vi "MOVE_ELEVATOR_TO_TARGET.vi"(10 "argv":string[](array[string]), 11 "args":u8) -> ()   [LabVIEW 2014]
uses:
  Robot Global Data.vi
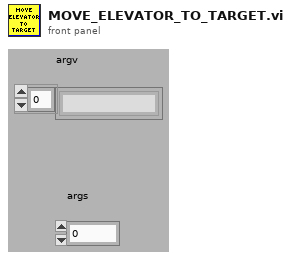
[diagram p1: front panel]
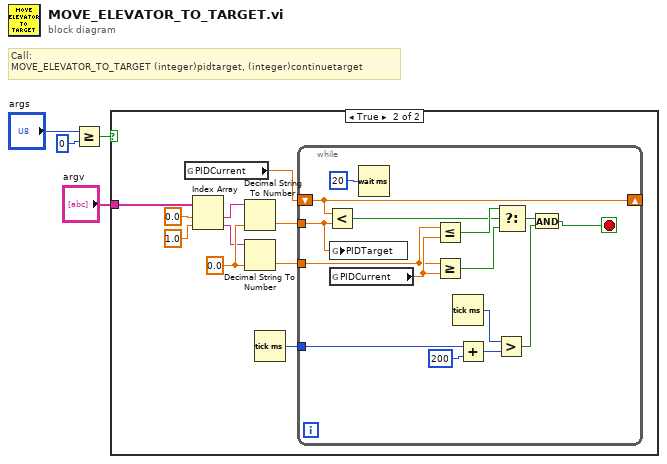
[diagram p0: block diagram]
diagram:
  # "Call:\nMOVE_ELEVATOR_TO_TARGET (integer)pidtarget, (integer)continuetarget"
  n1 = Greater Or Equal?(x="args", y=u8 0) -> (x >= y?=w4:bool)
  n2 = case shown="True" w4 {
    tunnel: "argv" -> [_ w11]
    frame False {
    }
    frame True {
      w6 = 0.0
      n3 = global read "OriginalPIDCurrent" "PIDCurrent"() -> (w13:dbl)
      n4 = Index Array(array=w11, index #1=0.0 ("default (0 I32)"), index #2=1.0 ("default (0 I32)")) -> (element #1=w9:string, element #2=w5:string)
      n5 = Decimal String To Number(string=w9, default (0L)=w6) -> (number=w8:dbl)  [unwired: 1 in, 1 out]
      n6 = Decimal String To Number(string=w5, default (0L)=w6) -> (number=w7:dbl)  [unwired: 1 in, 1 out]
      n7 = Tick Count (ms)() -> (millisecond timer value=w14:u32)
      n8 = while {
        tunnel: w8 -> [w19]
        tunnel: w14 -> [w16]
        tunnel: w7 -> [w18]
        shift-right: [w26] -> _
        shift-left: w13 -> [w26]
        stop <- w15 stop-if-true
        n9 = Less?(x=w26, y=w19) -> (x < y?=w21:bool)
        n10 = global write "Robot Global Data.vi" "PIDTarget"(w19) -> ()
        n11 = global read "OriginalPIDCurrent" "PIDCurrent"() -> (w20:dbl)
        n12 = Wait (ms)(milliseconds to wait=u32 20 ("millisecond multiple")) -> ()  [unwired: 1 out]
        n13 = Less Or Equal?(x=w18, y=w20) -> (x <= y?=w25:bool)
        n14 = Greater Or Equal?(x=w18, y=w20) -> (x >= y?=w24:bool)
        n15 = Tick Count (ms)() -> (millisecond timer value=w17:u32)
        n16 = Add(x=w16, y=u32 200) -> (x+y=w28:u32)
        n17 = Greater?(x=w17, y=w28) -> (0:w23:bool)
        n18 = Select(t=w25, s=w21, f=w24) -> (s? t:f=w22:bool)
        n19 = And(x=w22, y=w23) -> (x .and. y?=w15:bool)
      }
    }
  }
